vi "Increment Counter and Compute CRC.vi"(8 "error in (no error)":errorcluster, 11 "Frame In":T1 {"CRC" format="%08x"; "Frame Header"."Options" format="%016b"; "Frame Header"."Time" format="%^<%I:%M:%S%3u %p\n%m/%d/%Y %Z>T"; "Frame Header"."Sync" format="%08x"}) -> (0 "error out":errorcluster, 3 "Frame Out":T1 {"CRC" format="%08x"; "Frame Header"."Options" format="%016b"; "Frame Header"."Time" format="%^<%I:%M:%S%3u %p\n%m/%d/%Y %Z>T"; "Frame Header"."Sync" format="%08x"})   [LabVIEW 2021]
uses:
  Type Definitions/Data Frame.ctl
  Type Definitions/Data Frame Header.ctl
  Type Definitions/Payload Class.ctl
  Type Definitions/Device.ctl
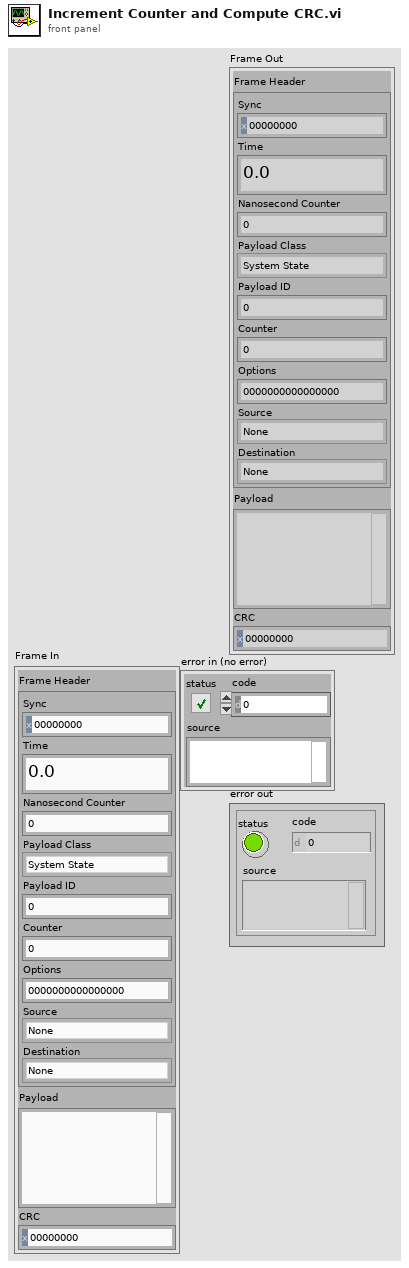
[diagram p1: front panel]
types:
  T1 = typedef "Data Frame.ctl" = cluster{"Frame Header":T2, "Payload":string, "CRC":u32}
  T2 = typedef "Data Frame Header.ctl" = cluster{"Sync":u32, "Time":dbl, "Nanosecond Counter":i64, "Payload Class":T3, "Payload ID":u16, "Counter":i32, "Options":u32, "Source":T4, "Destination":T4}
  T3 = typedef "Payload Class.ctl" = enum16{"System State", "Parameters", "Metadata", "Software Monitor", "Data", "Commands"}
  T4 = typedef "Device.ctl" = enum32{"None", "Exec", "Aux1", "Aux2", "Aux3"}
  T5 = cluster{"Sync":u32, "Time":dbl, "Nanosecond Counter":i64, "Payload Class":T3, "Payload ID":u16, "Counter":i32, "Options":u32, "Source":T4, "Destination":T4, "Payload":string}
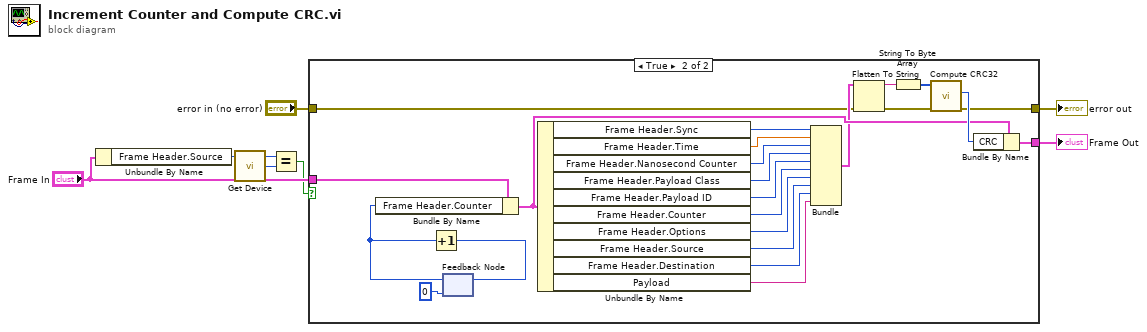
[diagram p0: block diagram]
diagram:
  n1 = Unbundle By Name("Frame In") -> ("Frame Header.Source"=w3:T4)
  n2 = call "Get Device.vi"() -> ("Device"=w2:T4)  [unwired: 5 in]
  n3 = Equal?(x=w3, y=w2) -> (x = y?=w1:bool)
  n4 = case shown="True" w1 {
    tunnel: [w8 w24] -> w7
    tunnel: "error in (no error)" -> [w9 w12]
    tunnel: [w9 w11] -> w5
    tunnel: "Frame In" -> [w8 w10]
    frame False {
    }
    frame True {
      n5 = feedback #1(u16 0 ("Counter")) -> (w28:u16)
      n6 = Bundle By Name(cluster=w10, "Frame Header.Counter"=w28) -> (w25:T1)
      n7 = Increment(x=w28) -> (x+1=w26:u16)
      n8 = feedback-in #1(w26) -> ()
      n9 = Unbundle By Name(w25) -> ("Frame Header.Sync"=w23:u32, "Frame Header.Time"=w22:dbl, "Frame Header.Nanosecond Counter"=w21:i64, "Frame Header.Payload Class"=w20:T3, "Frame Header.Payload ID"=w19:u16, "Frame Header.Counter"=w18:i32, "Frame Header.Options"=w17:u32, "Frame Header.Source"=w16:T4, "Frame Header.Destination"=w15:T4, "Payload"=w14:string)
      n10 = Bundle("Sync"=w23, "Time"=w22, "Nanosecond Counter"=w21, "Payload Class"=w20, "Payload ID"=w19, "Counter"=w18, "Options"=w17, "Source"=w16, "Destination"=w15, "Payload"=w14) -> (w13:T5)  [unwired: 1 in]
      n11 = Flatten To String(anything=w13, error in (no error)=w12) -> (data string=w32:string, error out=w31:errorcluster)  [unwired: 2 in, 1 out]
      n12 = String To Byte Array(string=w32) -> (unsigned byte array=w29:u8[])
      n13 = call "Compute CRC32.vi"("error in (no error)"=w31, "inputArray"=w29) -> ("error out"=w11:errorcluster, "CRC32Value"=w30:u32)  [unwired: 8 in]
      n14 = Bundle By Name(cluster=w25, "CRC"=w30) -> (w24:T1)
    }
  }
  "Frame Out" <- w7
  "error out" <- w5
